vi "SubVI3.vi"(2 "x":dbl, 3 "y":dbl) -> (9 "x+y":dbl)   [LabVIEW 2022 SP3]
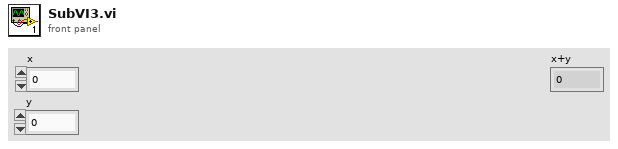
[diagram p1: front panel]
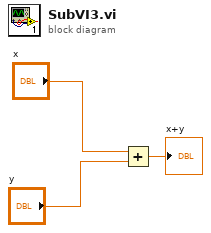
[diagram p0: block diagram]
diagram:
  n1 = Add(x="x", y="y") -> (x+y=→"x+y":dbl)
